vi "Panel DPT Voltage Labels.vi"(5 "Chanel List In":string, 7 "CDAQ?":bool, 9 "Label List In":string[](array[string])) -> (6 "Chanel List Out":string, 10 "Label List Out":string[](array[string]), 15 "Stream DC to File(out)?":bool)   [LabVIEW 2012]
uses:
  DPT Channel Label.ctl
  Global Test Variables DPT.vi
panel:
  in  "Stream DC to File?":bool
  in  "DC Voltages":T1[](array[typedef])=[{"Label"="", "Chan"="3021", "Rec"=FALSE, "TC Label"=""}, {"Label"="", "Chan"="3022", "Rec"=FALSE, "TC Label"=""}, {"Label"="", "Chan"="3023", "Rec"=FALSE, "TC Label"=""}, {"Label"="", "Chan"="3024", "Rec"=FALSE, "TC Label"=""}, {"Label"="", "Chan"="3025", "Rec"=FALSE, "TC Label"=""}, {"Label"="", "Chan"="3026", "Rec"=FALSE, "TC Label"=""}, {"Label"="", "Chan"="3027", "Rec"=FALSE, "TC Label"=""}, {"Label"="", "Chan"="3028", "Rec"=FALSE, "TC Label"=""}]
  in  "stop":bool
  in  "AC Voltages":T1[](array[typedef])=[{"Label"="", "Chan"="3001", "Rec"=FALSE, "TC Label"=""}, {"Label"="", "Chan"="3002", "Rec"=FALSE, "TC Label"=""}, {"Label"="", "Chan"="3003", "Rec"=FALSE, "TC Label"=""}, {"Label"="", "Chan"="3004", "Rec"=FALSE, "TC Label"=""}, {"Label"="", "Chan"="3005", "Rec"=FALSE, "TC Label"=""}, {"Label"="", "Chan"="3006", "Rec"=FALSE, "TC Label"=""}, {"Label"="", "Chan"="3007", "Rec"=FALSE, "TC Label"=""}, {"Label"="", "Chan"="3008", "Rec"=FALSE, "TC Label"=""}]
  # "Note that the channels are hiddent in the \ncontrol typedef. so that the user cannot change them."
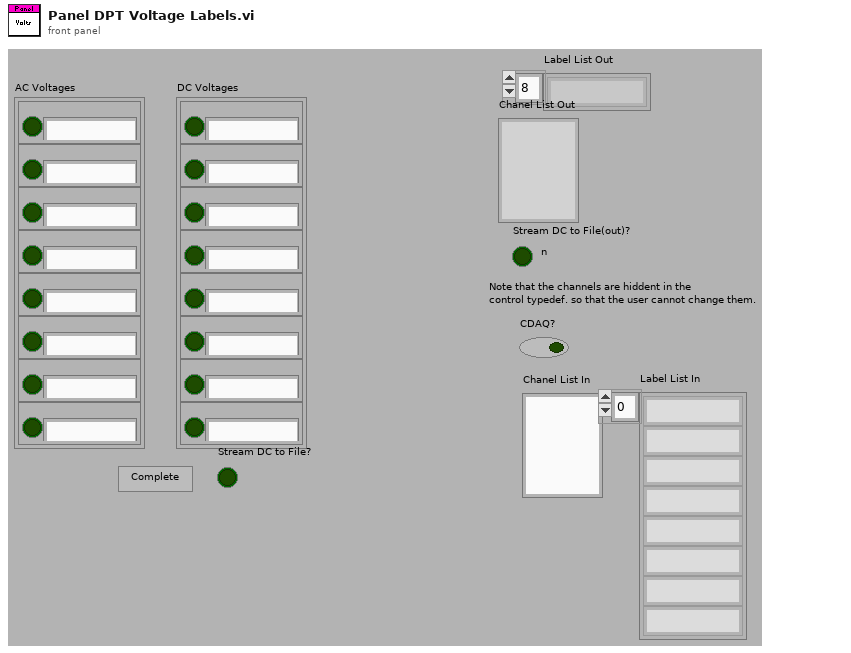
[diagram p1: front panel]
types:
  T1 = typedef "DPT Channel Label.ctl" = cluster{"Label":string, "Chan":string, "Rec":bool, "TC Label":string}
  T2 = typedef "DPT Global Type.ctl" = cluster{"Test Setup":cluster{"RH Resistor":dbl, "Temp Cal":dbl, "Temp Coeff":dbl, "Power On Threshold":dbl, "MA Filter Size":i32, "Weight Offset":dbl, "Temp Resistor":dbl, "Gas Enabled":bool, "Gas P. Resistor":dbl, "Scale Com":dbl, "W. Samps":i32, "Temp4mA Val":dbl, "Temp20mA Val":dbl, "RH4mA Val":dbl, "RH20mA Val":dbl, "GPres4mA Val":dbl, "Gpres20mA Val":dbl, "Smoothing":bool, "CDAQ":bool, "34970":bool, "34980":bool, "RH-IP":string, "RH-IP2":string, "RH-IP3":string, "CompVolume":dbl, "T45_Coeff.":dbl}, "Agilent Setup":cluster{"Scale Channel":string, "TC Channels":string, "VDC Discrete Channels":string, "RH Chan":string, "Temp Chan":string, "Tscale Channel":string, "RDB Channel":string, "Gas Temperature":string, "Gas Pressure":string, "Barometric Pressure":string, "Gas Feedback Chan":string}, "Directories":cluster{"Work File Directory":path, "Save File Directory":path, "Library Directory":path, "Data Backup Directory":path, "Data Backup Dir Fail":path, "Lab Directory":path}, "Test Information":cluster{"Model:":string, "Temperature:":string, "Engineer:":string, "Technician:":string, "Comments:":string, "Lab ID:":string, "TR Number:":string, "Test Number:":string, "Test Station:":string, "Empty Dryer Cold Weight:":dbl, "Serial Number:":string, "Build:":string, "Dryer Type":string, "Humidity":string, "Test Title per TR:":string}, "cDAQ Array Locations":cluster{"Scale Channel":string, "TC Channels":string, "VDC Discrete Channel":string, "RH Chan":string, "Temp Chan":string, "Tscale Channel":string, "RDB Channel":string, "Gas Temperature":string, "Gas Pressure":string, "Barometric Pressure":string, "Gas Feedback Chan":string}}
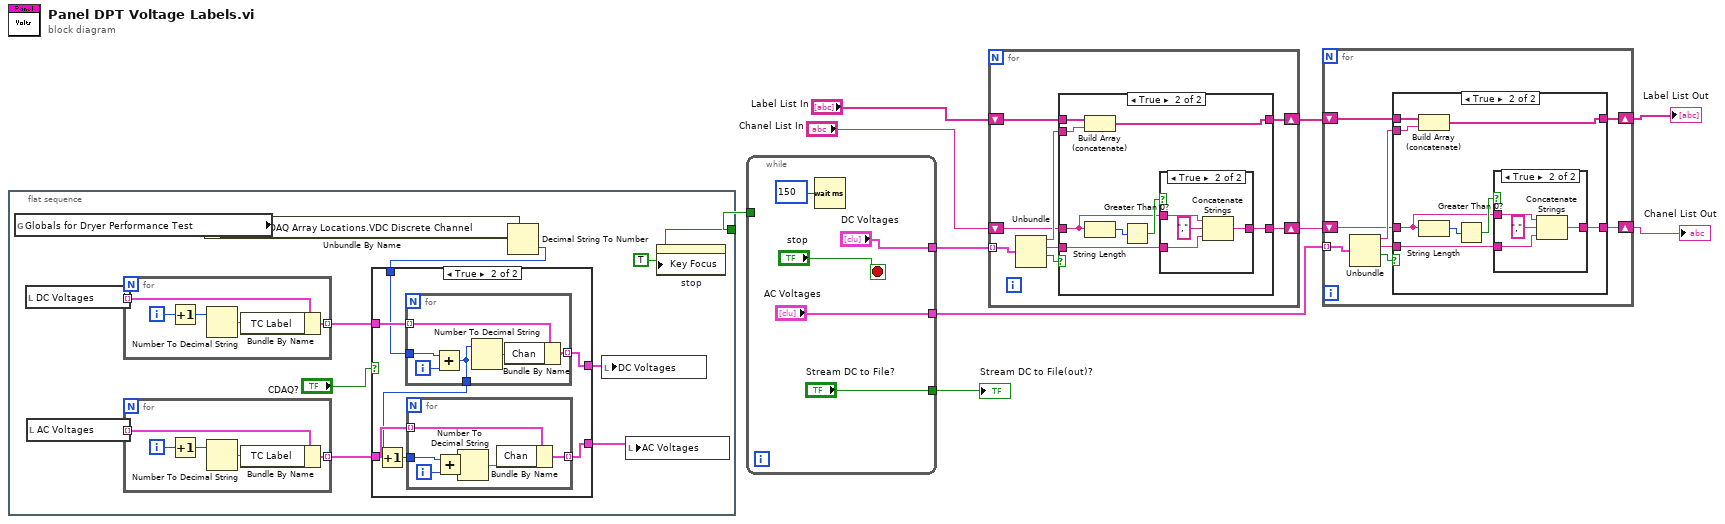
[diagram p0: block diagram]
diagram:
  n1 = flat-sequence {
    tunnel: [w21] -> w2
    frame #0 {
      w21 = TRUE ("Key Focus")
      n2 = global read "Global Test Variables DPT.vi" "Globals for Dryer Performance Test"() -> (w12:T2)
      n3 = local read "DC Voltages"() -> (w19:T1[])
      n4 = local read "AC Voltages"() -> (w20:T1[])
      n5 = for {
        tunnel: w19 -> [w47] mode=indexing
        tunnel: [w46] -> w16 mode=indexing
        i -> [w45]
        n6 = Increment(x=w45) -> (x+1=w44:i32)
        n7 = Number To Decimal String(number=w44) -> (decimal integer string=w43:string)  [unwired: 1 in]
        n8 = Bundle By Name(cluster=w47, "TC Label"=w43) -> (w46:T1)
      }
      n9 = for {
        tunnel: w20 -> [w52] mode=indexing
        tunnel: [w51] -> w14 mode=indexing
        i -> [w50]
        n10 = Increment(x=w50) -> (x+1=w49:i32)
        n11 = Number To Decimal String(number=w49) -> (decimal integer string=w48:string)  [unwired: 1 in]
        n12 = Bundle By Name(cluster=w52, "TC Label"=w48) -> (w51:T1)
      }
      n13 = Unbundle By Name(w12) -> ("cDAQ Array Locations.VDC Discrete Channel"=w13:string)
      n14 = Decimal String To Number(string=w13) -> (number=w11:i32)  [unwired: 2 in, 1 out]
      n15 = case shown="True" "CDAQ?" {
        tunnel: [w23 w28] -> w17
        tunnel: w16 -> [w23 w30]
        tunnel: [w22 w27] -> w15
        tunnel: w14 -> [w22 w26]
        tunnel: w11 -> [_ w29]
        frame False {
        }
        frame True {
          n16 = for {
            tunnel: w30 -> [w42] mode=indexing
            tunnel: w29 -> [w40]
            tunnel: [w38] -> w28 mode=indexing
            tunnel: [w37] -> w25
            i -> [w41]
            n17 = Add(x=w40, y=w41) -> (x+y=w37:i32)
            n18 = Number To Decimal String(number=w37) -> (decimal integer string=w39:string)  [unwired: 1 in]
            n19 = Bundle By Name(cluster=w42, "Chan"=w39) -> (w38:T1)
          }
          n20 = Increment(x=w25) -> (x+1=w24:i32)
          n21 = for {
            tunnel: w26 -> [w36] mode=indexing
            tunnel: w24 -> [w34]
            tunnel: [w31] -> w27 mode=indexing
            i -> [w35]
            n22 = Add(x=w34, y=w35) -> (x+y=w32:i32)
            n23 = Number To Decimal String(number=w32) -> (decimal integer string=w33:string)  [unwired: 1 in]
            n24 = Bundle By Name(cluster=w36, "Chan"=w33) -> (w31:T1)
          }
        }
      }
      n25 = local write "DC Voltages"(w17) -> ()
      n26 = local write "AC Voltages"(w15) -> ()
      n27 = property on="stop" class="Bool"("Key Focus"=w21) -> ()  [unwired: 2 in, 2 out]
    }
  }
  n28 = while {
    tunnel: ["DC Voltages"] -> w10
    tunnel: ["AC Voltages"] -> w5
    tunnel: w2 -> [_]
    tunnel: ["Stream DC to File?"] -> w1
    stop <- "stop" stop-if-true
    n29 = Wait (ms)(milliseconds to wait=u32 150) -> ()  [unwired: 1 out]
  }
  "Stream DC to File(out)?" <- w1
  n30 = for {
    tunnel: w10 -> [w65] mode=indexing
    shift-right: [w61] -> w7
    shift-left: "Label List In" -> [w62]
    shift-right: [w59] -> w6
    shift-left: "Chanel List In" -> [w58]
    n31 = Unbundle(w65) -> ("Label"=w63:string, "Chan"=w60:string, "Rec"=w64:bool)  [unwired: 1 out]
    n32 = case shown="True" w64 {
      tunnel: w63 -> [_ w75]
      tunnel: w62 -> [w67 w74]
      tunnel: [w67 w73] -> w61
      tunnel: w58 -> [w66 w70]
      tunnel: w60 -> [_ w69]
      tunnel: [w66 w68] -> w59
      frame False {
      }
      frame True {
        n33 = Build Array (concatenate)(w74, w75) -> (w73:string[])
        n34 = String Length(string=w70) -> (length=w72:i32)
        n35 = Greater Than 0?(x=w72) -> (x > 0?=w71:bool)
        n36 = case shown="True" w71 {
          tunnel: w70 -> [_ w80]
          tunnel: w69 -> [w76 w78]
          tunnel: [w76 w77] -> w68
          frame False {
          }
          frame True {
            n37 = Concatenate Strings(w80, "," ("string"), w78) -> (w77:string)
          }
        }
      }
    }
  }
  n38 = for {
    tunnel: w5 -> [w88] mode=indexing
    shift-right: [w84] -> w4
    shift-left: w7 -> [w85]
    shift-right: [w82] -> w3
    shift-left: w6 -> [w81]
    n39 = Unbundle(w88) -> ("Label"=w86:string, "Chan"=w83:string, "Rec"=w87:bool)  [unwired: 1 out]
    n40 = case shown="True" w87 {
      tunnel: w86 -> [_ w98]
      tunnel: w85 -> [w90 w97]
      tunnel: [w90 w96] -> w84
      tunnel: w81 -> [w89 w93]
      tunnel: w83 -> [_ w92]
      tunnel: [w89 w91] -> w82
      frame False {
      }
      frame True {
        n41 = Build Array (concatenate)(w97, w98) -> (w96:string[])
        n42 = String Length(string=w93) -> (length=w95:i32)
        n43 = Greater Than 0?(x=w95) -> (x > 0?=w94:bool)
        n44 = case shown="True" w94 {
          tunnel: w93 -> [_ w103]
          tunnel: w92 -> [w99 w101]
          tunnel: [w99 w100] -> w91
          frame False {
          }
          frame True {
            n45 = Concatenate Strings(w103, "," ("string"), w101) -> (w100:string)
          }
        }
      }
    }
  }
  "Label List Out" <- w4
  "Chanel List Out" <- w3
